vi "Find Signals File.vi"(8 "error in":errorcluster, 10 "Application Directory":path, 11 "SLL in":refnum<class "SLL.lvclass">) -> (0 "error out":errorcluster, 3 "SLL out":refnum<class "SLL.lvclass">)   [LabVIEW 2023, in "SLL.lvlib" / "SLL.lvclass"]
uses:
  SLL.lvclass
  SLL.lvclass/SLL.ctl
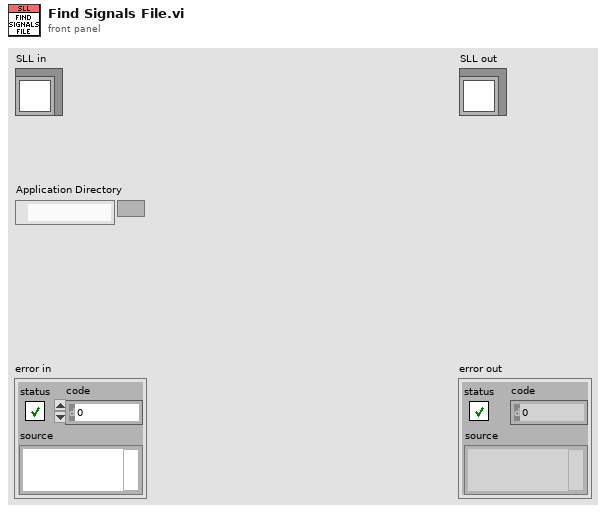
[diagram p1: front panel]
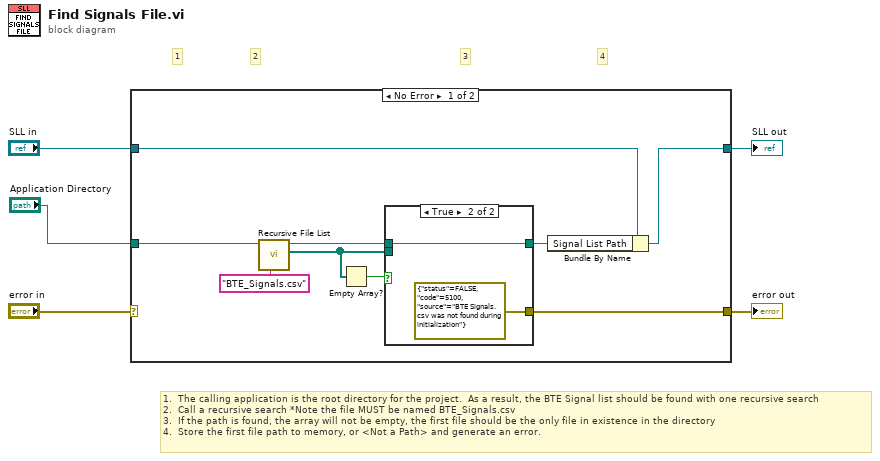
[diagram p0: block diagram]
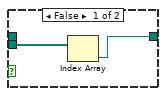
[diagram p2: hidden frame]
diagram:
  # "1.  The calling application is the root directory for the project.  As a result, the BTE Signal list should be found with one recursive search\n2.  Call a recursive search *Note the file MUST be named BTE_Signals.csv\n3.  If the path is found, the array will not be empty, the first file should be the only file in existence in the directory\n4.  Store the first file path to memory, or <Not a Path> and generate an error."
  # "4"
  # "3"
  # "2"
  # "1"
  n1 = case shown="No Error" "error in" {
    selector: "error in" -> [_ w20]
    tunnel: [w7 w20] -> w4
    tunnel: [w13 w19] -> w2
    tunnel: "SLL in" -> [w14 w19]
    tunnel: "Application Directory" -> [w6 _]
    frame No Error {
      n2 = call <vilib>:"Recursive File List.vi"("pattern"="BTE_Signals.csv", "Folder Path"=w6) -> ("All Files in Dir"=w9:path[], "dup Folder Path"=w10:path)  [unwired: 5 in, 3 out]
      n3 = Empty Array?(array=w9) -> (empty?=w11:bool)
      n4 = case shown="True" w11 {
        tunnel: w10 -> [_ w18]
        tunnel: w9 -> [w16 _]
        tunnel: [w15 w18] -> w8
        tunnel: [_ errorcluster {"status"=FALSE, "code"=5100, "source"="BTE Signals.csv was not found during initialization"} ("error constant")] -> w7
        frame False {
          n5 = Index Array(array=w16) -> (element=w15:path)  [unwired: 1 in]
        }
        frame True {
        }
      }
      n6 = Bundle By Name(cluster=w14, "Signal List Path"=w8) -> (w13:refnum<class "SLL.lvclass">)
    }
    frame Error {
    }
  }
  "error out" <- w4
  "SLL out" <- w2
